vi "ex_Read Lines From File.vi"(5 "convert eol? (no:F)":bool, 6 "[max characters per line]  (no limit:0)":i32, 8 "error in (not an error)":errorcluster, 9 "start of read offset (chars.:0 )":i32, 10 "number of lines (all:-1)":i32=-1, 11 "file path (dialog if empty)":path) -> (0 "error out":errorcluster, 1 "mark after read (chars.)":i32, 2 "line string":string, 3 "new file path (Not A Path if cancelled)":path, 4 "EOF?":bool)   [LabVIEW 2020]
doc: "LabVIEW no longer supports this VI. Use the Read from Text File function instead."
panel:
  in  "prompt":string="Choose file to read."
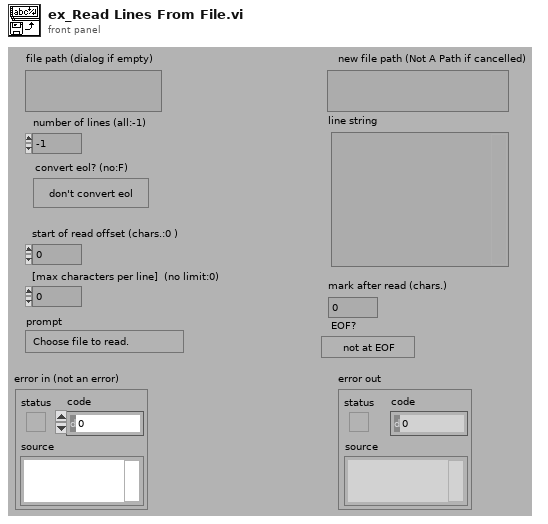
[diagram p1: front panel]
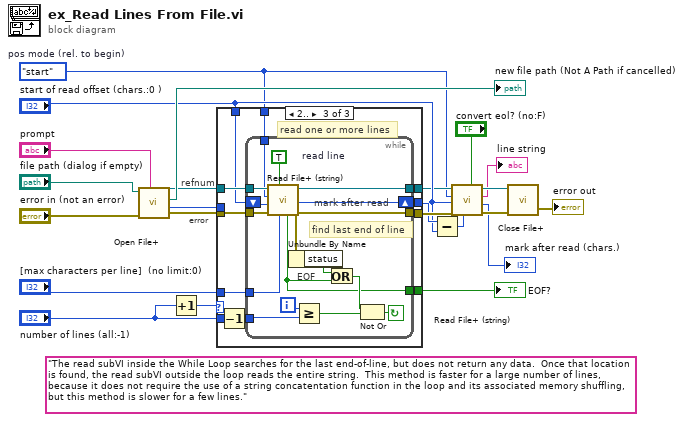
[diagram p0: block diagram]
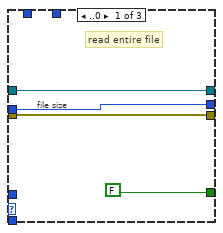
[diagram p2: hidden frame]
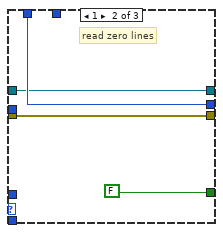
[diagram p3: hidden frame]
diagram:
  w4 = enum16{"start", "end", "current"}."start"  # pos mode (rel. to begin)
  (unwired) "The read subVI inside the While Loop searches for the last end-of-line, but does not return any data.  Once that location is found, the read subVI outside the loop reads the entire string.  This method is faster for a large number of lines, because it does not require the use of a string concatentation function in the loop and its associated memory shuffling, but this method is slower for a few lines."
  # "error"
  # "refnum"
  n1 = call <vilib>:"Open File+.vi"("prompt"="prompt", "error in (not an error)"="error in (not an error)", "file path (\" \")"="file path (dialog if empty)") -> ("error out"=w11:errorcluster, "file size (bytes)"=w8:i32, "file path"=→"new file path (Not A Path if cancelled)":path, "refnum"=w10:refnum<file>)  [unwired: 5 in]
  n2 = Increment(x="number of lines (all:-1)") -> (x+1=w13:i32)
  n3 = case shown="2.." w13 {
    tunnel: [w27 w30 w42] -> w15
    tunnel: [w26 w31 w41] -> w14
    tunnel: "number of lines (all:-1)" -> [_ _ w40]
    tunnel: "[max characters per line]  (no limit:0)" -> [_ _ w39]
    tunnel: w11 -> [w27 w30 w38]
    tunnel: w10 -> [w25 w29 w37]
    tunnel: "start of read offset (chars.:0 )" -> [_ w31 w36]
    tunnel: w4 -> [_ _ w35]
    tunnel: w8 -> [w26 _ _]
    tunnel: [w25 w29 w34] -> w7
    tunnel: [FALSE FALSE w33] -> w6
    frame ..0 {
      # "file size"
      # "read entire file"
    }
    frame 1 {
      # "read zero lines"
    }
    frame 2.. {
      # "read one or more lines"
      n4 = Decrement(x=w40) -> (x-1=w32:i32)
      n5 = while {
        tunnel: [w44] -> w33
        tunnel: w35 -> [w49]
        tunnel: w38 -> [w51]
        tunnel: w39 -> [w52]
        tunnel: [w47] -> w42
        tunnel: w37 -> [w54]
        tunnel: [w55] -> w34
        tunnel: w32 -> [w43]
        shift-left: w36 -> [w56]
        shift-right: [w58] -> w41
        i -> [w57]
        stop <- w50 continue-if-true
        w46 = TRUE  # read line
        # "mark after read"
        # "find last end of line"
        # "EOF"
        n6 = call <vilib>:"Read File+ (string).vi"("count"=w52, "line mode (characters:F)"=w46, "error in (no error)"=w51, "pos offset (bytes:0)"=w56, "pos mode (rel. to current:2)"=w49, "refnum"=w54) -> ("error out"=w47:errorcluster, "mark after read (bytes)"=w58:i32, "dup refnum"=w55:refnum<file>, "EOF?"=w44:bool)  [unwired: 1 in, 1 out]
        n7 = Unbundle By Name(w47) -> ("status"=w45:bool)
        n8 = Greater Or Equal?(x=w57, y=w43) -> (x >= y?=w53:bool)
        n9 = Or(x=w45, y=w44) -> (x .or. y?=w48:bool)
        n10 = Not Or(1:w53, 2:w48) -> (0:w50:bool)
      }
    }
  }
  "EOF?" <- w6
  n11 = Subtract(x=w14, y="start of read offset (chars.:0 )") -> (x-y=w20:i32)
  n12 = call <vilib>:"Read File+ (string).vi"("convert eol? (no:F)"="convert eol? (no:F)", "count"=w20, "error in (no error)"=w15, "pos offset (bytes:0)"="start of read offset (chars.:0 )", "pos mode (rel. to current:2)"=w4, "refnum"=w7) -> ("error out"=w21:errorcluster, "mark after read (bytes)"=→"mark after read (chars.)":i32, "string"=→"line string":string, "dup refnum"=w22:refnum<file>)  [unwired: 1 in, 1 out]
  n13 = call <vilib>:"Close File+.vi"("error in (no error)"=w21, "refnum"=w22) -> ("error out"=→"error out":errorcluster)  [unwired: 3 in, 2 out]
